vi "Check Readable String.vi"(1 "String":string) -> (0 "Valid":bool)   [LabVIEW 2020, in "Protobuf RAW.lvlib" / "string.lvclass"]
uses:
  string.lvclass
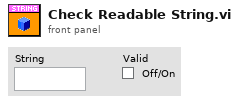
[diagram p1: front panel]
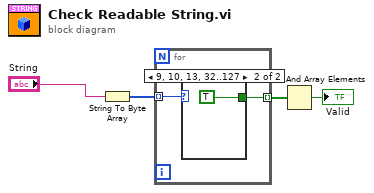
[diagram p0: block diagram]
diagram:
  n1 = String To Byte Array(string="String") -> (unsigned byte array=w2:u8[])
  n2 = for {
    tunnel: w2 -> [w6] mode=indexing
    tunnel: [w5] -> w3 mode=indexing
    n3 = case shown="9, 10, 13, 32..127" w6 {
      tunnel: [_ TRUE] -> w5
      frame 0, Default {
      }
      frame 9, 10, 13, 32..127 {
      }
    }
  }
  n4 = And Array Elements(Boolean array=w3) -> (logical AND=→"Valid":bool)
